vi "Write To TDMS File.vi"(7 "Data Cluster In":T1, 8 "error in (no error)":errorcluster, 11 "Releative Time":dbl format="%#_13g") -> (0 "error out":errorcluster, 5 "Data Cluster Out":T1)   [LabVIEW 2021, in "RT-TDMS-Logging.lvlib"]
uses:
  RT-TDMS-Logging.lvlib
  Module Data--cluster.ctl
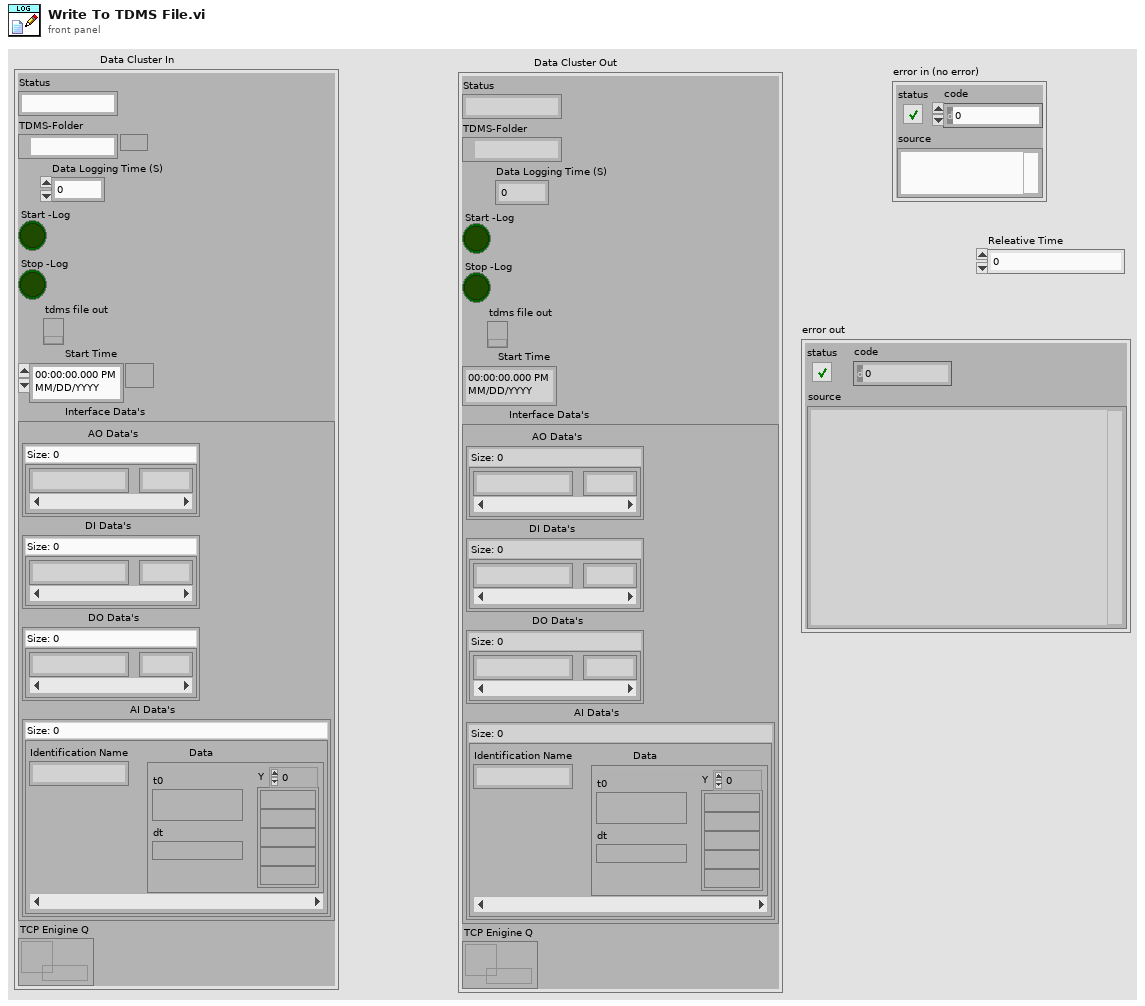
[diagram p1: front panel]
types:
  T1 = typedef "RT-TDMS-Logging.lvlib/Module Data--cluster.ctl" = cluster{"Status":string, "TDMS-Folder":path, "Data Logging Time (S)":dbl, "Start -Log":bool, "Stop -Log":bool, "tdms file out":refnum<k34>, "Start Time":timestamp, "Interface Data's":cluster{"AO Data's":map{string, dbl}, "DI Data's":map{string, i16}, "DO Data's":map{string, i16}, "AI Data's":map{string, waveform(dbl)}}, "TCP Enigine Q":refnum<queue>}
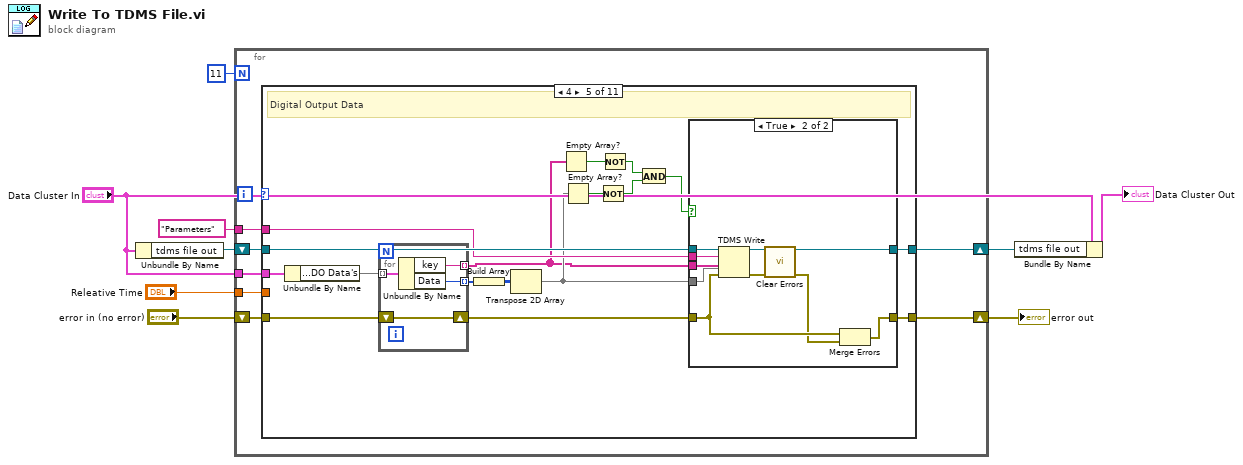
[diagram p0: block diagram]
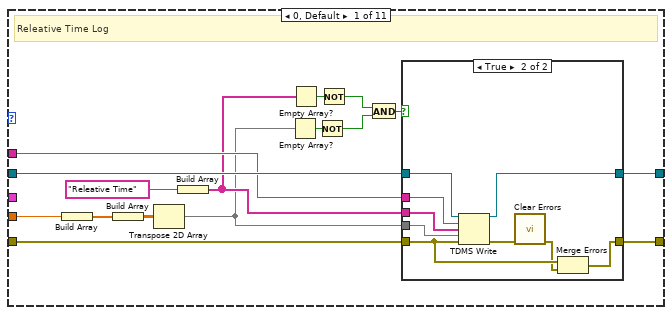
[diagram p2: hidden frame]
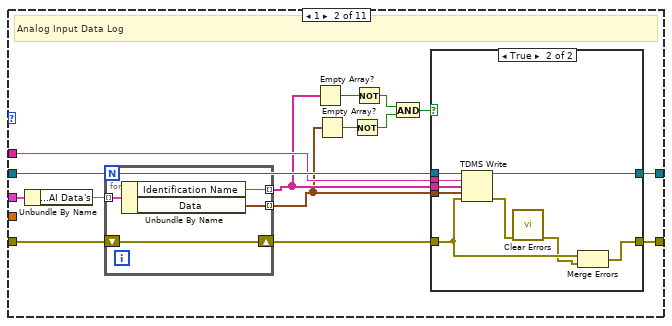
[diagram p4: hidden frame]
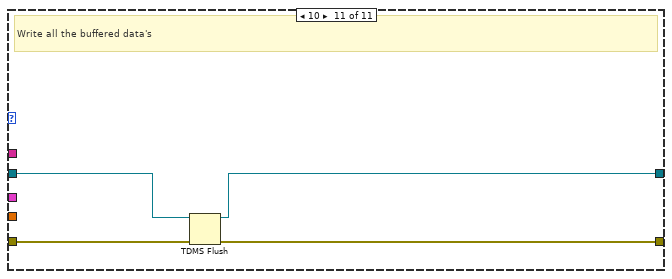
[diagram p14: hidden frame]
diagram:
  n1 = Unbundle By Name("Data Cluster In") -> ("tdms file out"=w9:refnum<k34>)
  n2 = for {
    N: 11 -> [_]
    shift-right: [w16] -> w8
    shift-left: w9 -> [w17]
    tunnel: "Parameters" -> [w15]
    tunnel: "Data Cluster In" -> [w13]
    shift-right: [w11] -> w4
    shift-left: "error in (no error)" -> [w12]
    tunnel: "Releative Time" -> [w10]
    i -> [w14]
    n3 = case shown="4" w14 {
      tunnel: w17 -> [w31 w59 w76 w78 w95 w112 w114 w116 w118 w120 w124]
      tunnel: [w30 w58 w76 w78 w93 w112 w114 w116 w118 w120 w123] -> w16
      tunnel: w15 -> [w29 w57 _ _ w94 _ _ _ _ _ _]
      tunnel: w13 -> [_ w56 _ _ w91 _ _ _ _ _ _]
      tunnel: w12 -> [w33 w54 w75 w77 w86 w111 w113 w115 w117 w119 w122]
      tunnel: [w32 w55 w75 w77 w92 w111 w113 w115 w117 w119 w121] -> w11
      tunnel: w10 -> [w25 _ _ _ _ _ _ _ _ _ _]
      frame 0, Default {
        # "Releative Time Log"
        n4 = Build Array(w25) -> (w26:dbl[])
        n5 = Build Array(w26) -> (w27:dbl[][])
        n6 = Transpose 2D Array(2D array=w27) -> (transposed array=w18:dbl[][])
        n7 = Build Array("Releative Time") -> (w19:string[])
        n8 = Empty Array?(array=w18) -> (empty?=w23:bool)
        n9 = Empty Array?(array=w19) -> (empty?=w24:bool)
        n10 = Not(x=w23) -> (.not. x?=w21:bool)
        n11 = Not(x=w24) -> (.not. x?=w22:bool)
        n12 = And(x=w22, y=w21) -> (x .and. y?=w20:bool)
        n13 = case shown="True" w20 {
          tunnel: w33 -> [w34 w39]
          tunnel: [w34 w37] -> w32
          tunnel: w31 -> [w35 w44]
          tunnel: [w35 w43] -> w30
          tunnel: w29 -> [_ w42]
          tunnel: w19 -> [_ w41]
          tunnel: w18 -> [_ w40]
          frame False {
          }
          frame True {
            n14 = TDMS Write(0:w44, 5:w42, 7:w41, 9:w40, 11:w39) -> (4:w43:refnum<k34>, 15:w38:errorcluster)  [unwired: 1 in, 2 out]
            n15 = call <vilib>:"Clear Errors.vi"("error in (no error)"=w38) -> ("error out"=w36:errorcluster)  [unwired: 5 in, 1 out]
            n16 = Merge Errors(w39, w36) -> (w37:errorcluster)
          }
        }
      }
      frame 1 {
        # "Analog Input Data Log"
        n17 = Unbundle By Name(w56) -> ("Interface Data's.AI Data's"=w52:map{string, waveform(dbl)})
        n18 = for {
          tunnel: w52 -> [w74] mode=indexing
          tunnel: [w73] -> w50 mode=indexing
          tunnel: [w72] -> w51 mode=indexing
          shift-right: [w71] -> w53
          shift-left: w54 -> [w71]
          n19 = Unbundle By Name(w74) -> ("Identification Name"=w72:string, "Data"=w73:waveform(dbl))
        }
        n20 = Empty Array?(array=w51) -> (empty?=w49:bool)
        n21 = Empty Array?(array=w50) -> (empty?=w48:bool)
        n22 = Not(x=w48) -> (.not. x?=w45:bool)
        n23 = Not(x=w49) -> (.not. x?=w46:bool)
        n24 = And(x=w46, y=w45) -> (x .and. y?=w47:bool)
        n25 = case shown="True" w47 {
          tunnel: w59 -> [w61 w70]
          tunnel: [w61 w69] -> w58
          tunnel: w57 -> [_ w68]
          tunnel: [w60 w63] -> w55
          tunnel: w53 -> [w60 w65]
          tunnel: w50 -> [_ w67]
          tunnel: w51 -> [_ w66]
          frame False {
          }
          frame True {
            n26 = TDMS Write(0:w70, 5:w68, 7:w66, 9:w67, 11:w65) -> (4:w69:refnum<k34>, 15:w64:errorcluster)  [unwired: 1 in, 2 out]
            n27 = call <vilib>:"Clear Errors.vi"("error in (no error)"=w64) -> ("error out"=w62:errorcluster)  [unwired: 5 in, 1 out]
            n28 = Merge Errors(w65, w62) -> (w63:errorcluster)
          }
        }
      }
      frame 2 {
      }
      frame 3 {
      }
      frame 4 {
        # "Digital Output Data"
        n29 = Unbundle By Name(w91) -> ("Interface Data's.DO Data's"=w89:map{string, i16})
        n30 = for {
          tunnel: w89 -> [w110] mode=indexing
          tunnel: [w109] -> w88 mode=indexing
          tunnel: [w108] -> w79 mode=indexing
          shift-right: [w107] -> w87
          shift-left: w86 -> [w107]
          n31 = Unbundle By Name(w110) -> ("key"=w108:string, "Data"=w109:i16)
        }
        n32 = Build Array(w88) -> (w90:i16[][])
        n33 = Transpose 2D Array(2D array=w90) -> (transposed array=w80:i16[][])
        n34 = Empty Array?(array=w79) -> (empty?=w85:bool)
        n35 = Empty Array?(array=w80) -> (empty?=w84:bool)
        n36 = Not(x=w84) -> (.not. x?=w82:bool)
        n37 = Not(x=w85) -> (.not. x?=w83:bool)
        n38 = And(x=w83, y=w82) -> (x .and. y?=w81:bool)
        n39 = case shown="True" w81 {
          tunnel: w95 -> [w97 w106]
          tunnel: w94 -> [_ w105]
          tunnel: [w97 w104] -> w93
          tunnel: [w96 w99] -> w92
          tunnel: w80 -> [_ w103]
          tunnel: w79 -> [_ w102]
          tunnel: w87 -> [w96 w101]
          frame False {
          }
          frame True {
            n40 = TDMS Write(0:w106, 5:w105, 7:w102, 9:w103, 11:w101) -> (4:w104:refnum<k34>, 15:w100:errorcluster)  [unwired: 1 in, 2 out]
            n41 = call <vilib>:"Clear Errors.vi"("error in (no error)"=w100) -> ("error out"=w98:errorcluster)  [unwired: 5 in, 1 out]
            n42 = Merge Errors(w101, w98) -> (w99:errorcluster)
          }
        }
      }
      frame 5 {
      }
      frame 6 {
      }
      frame 7 {
      }
      frame 8 {
      }
      frame 9 {
      }
      frame 10 {
        # "Write all the buffered data's"
        n43 = TDMS Flush(4:w122, 7:w124) -> (0:w121:errorcluster, 3:w123:refnum<k34>)
      }
    }
  }
  "error out" <- w4
  n44 = Bundle By Name(cluster="Data Cluster In", "tdms file out"=w8) -> (→"Data Cluster Out":T1)
